vi "ESP301 Home.vi"(5 "Axe Inv":bool, 6 "Input Units":i8(ring) items=["mm", "ps"], 7 "ESP301Ref":T1, 8 "error in":errorcluster, 9 "Axis":i8(ring)=1 items=["Axis 1"=1, "Axis 2"=2, "Axis 3"=3], 11 "VISA Rsrc":refnum<visa-resource-name>="GPIB0::7::INSTR") -> (0 "error out":errorcluster)   [LabVIEW 2019]
uses:
  <userlib>/ESP300/ESP300 GotoState.ctl
  <userlib>/GenProg/WritebyRefNum.vi
panel:
  out "Position":dbl=0.5
  out "Move Done":bool
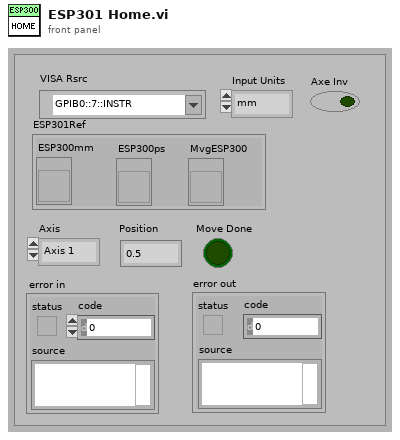
[diagram p1: front panel]
types:
  T1 = cluster{"ESP300mm":refnum<vi>, "ESP300ps":refnum<vi>, "MvgESP300":refnum<vi>}
  T2 = typedef "ESP300 GotoState.ctl" = enum16{"send command", "read position", "check status", "end"}
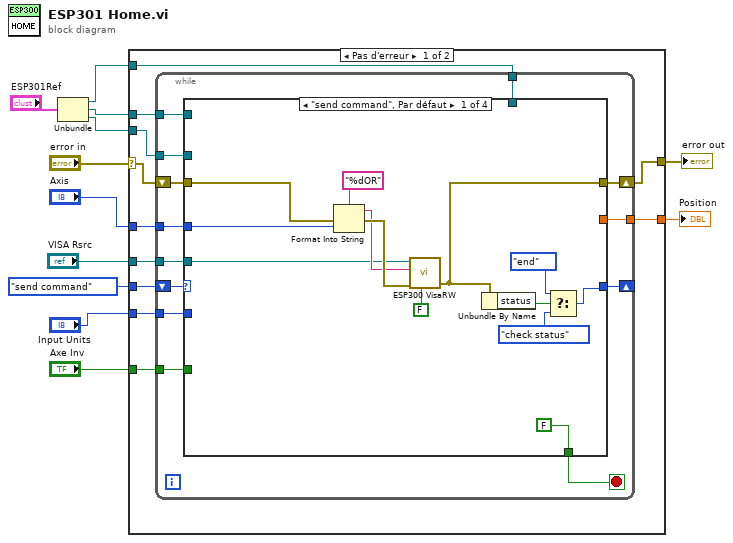
[diagram p0: block diagram]
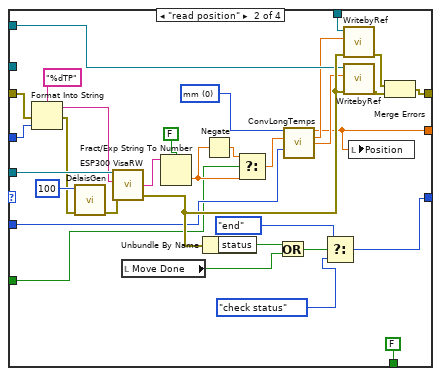
[diagram p2: hidden frame]
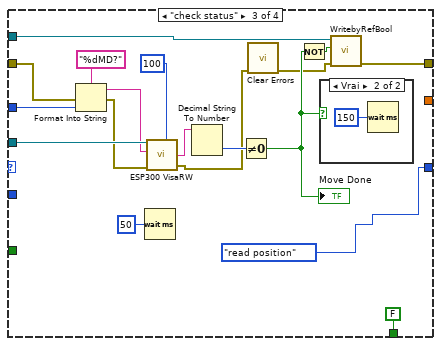
[diagram p3: hidden frame]
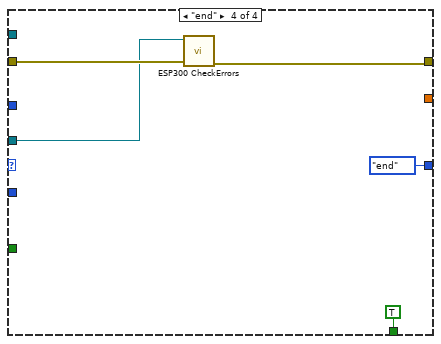
[diagram p5: hidden frame]
diagram:
  n1 = Unbundle("ESP301Ref") -> ("ESP300mm"=w3:refnum<vi>, "ESP300ps"=w5:refnum<vi>, "MvgESP300"=w4:refnum<vi>)
  n2 = case shown="Pas d'erreur" "error in" {
    selector: "error in" -> [w21 w106]
    tunnel: "Axis" -> [w23 _]
    tunnel: [w20 w106] -> w10
    tunnel: ESP300_GotoState."send command" ("Énum") -> [w22 _]
    tunnel: "VISA Rsrc" -> [w19 _]
    tunnel: w4 -> [w18 _]
    tunnel: "Input Units" -> [w17 _]
    tunnel: w3 -> [w16 _]
    tunnel: w5 -> [w15 _]
    tunnel: "Axe Inv" -> [w14 _]
    tunnel: [w13 _] -> w1
    frame No Error {
      n3 = while {
        tunnel: w23 -> [w36]
        shift-right: [w32] -> w20
        shift-left: w21 -> [w34]
        tunnel: w19 -> [w33]
        shift-right: [w30] -> _
        shift-left: w22 -> [w35]
        tunnel: w18 -> [w29]
        tunnel: w17 -> [w28]
        tunnel: w16 -> [w27]
        tunnel: w15 -> [w26]
        tunnel: w14 -> [w25]
        tunnel: [w24] -> w13
        stop <- w31 stop-if-true
        n4 = case shown="\"send command\", Par défaut" w35 {
          tunnel: w36 -> [w48 w79 w97 _]
          tunnel: w34 -> [w47 w78 w96 w103]
          tunnel: w33 -> [w44 w81 w99 w101]
          tunnel: [w41 w62 w87 w102] -> w32
          tunnel: [FALSE FALSE FALSE TRUE] -> w31
          tunnel: [w38 w71 ESP300_GotoState."read position" ("Énum") ESP300_GotoState."end" ("Énum")] -> w30
          tunnel: w29 -> [_ _ w89 _]
          tunnel: w28 -> [_ w55 _ _]
          tunnel: w27 -> [_ w60 _ _]
          tunnel: w26 -> [_ w59 _ _]
          tunnel: w25 -> [_ w51 _ _]
          tunnel: [_ w50 _ _] -> w24
          frame "send command", Default {
            n5 = Format Into String(format string="%dOR", error in=w47, w48) -> (resulting string=w45:string, error out=w46:errorcluster)  [unwired: 1 in]
            n6 = call <userlib>:"ESP300 VisaRW.vi"("Lecture?(T)"=FALSE, "error in (no error)"=w46, "ChaineCom"=w45, "VISA Rsrc"=w44) -> ("error out"=w41:errorcluster)  [unwired: 3 in, 3 out]
            n7 = Unbundle By Name(w41) -> ("status"=w40:bool)
            n8 = Select(t=ESP300_GotoState."end" ("Énum"), s=w40, f=ESP300_GotoState."check status" ("Énum")) -> (s? t:f=w38:T2)
          }
          frame "read position" {
            w58 = i8 0 items=["mm", "ps"] ("Input Units")
            n9 = Format Into String(format string="%dTP", error in=w78, w79) -> (resulting string=w77:string, error out=w66:errorcluster)  [unwired: 1 in]
            n10 = call "DélaisGen.vi"("error in (no error)"=w66, "ms To Wait"=u32 100 ("milliseconds to wait")) -> ("error out"=w67:errorcluster)  [unwired: 9 in]
            n11 = call <userlib>:"ESP300 VisaRW.vi"("error in (no error)"=w67, "ChaineCom"=w77, "VISA Rsrc"=w81) -> ("error out"=w63:errorcluster, "ChaineRep"=w76:string)  [unwired: 4 in, 2 out]
            n12 = local read "Move Done"() -> (w65:bool)
            n13 = Fract/Exp String To Number(use system decimal point (T)=FALSE ("utiliser le séparateur décimal du système (V)"), string=w76) -> (number=w53:dbl)  [unwired: 2 in, 1 out]
            n14 = Unbundle By Name(w63) -> ("status"=w70:bool)
            n15 = Negate(x=w53) -> (-x=w54:dbl)
            n16 = Select(t=w54, s=w51, f=w53) -> (s? t:f=w52:dbl)
            n17 = Or(x=w70, y=w65) -> (x .or. y?=w69:bool)
            n18 = call <userlib>:"ConvLongTemps.vi"("Input Units"=w58, "Units Input"=w52, "Output Units"=w55) -> ("Units Output"=w50:dbl, "Units mm"=w57:dbl, "Units ps"=w56:dbl)  [unwired: 9 in, 1 out]
            n19 = Select(t=ESP300_GotoState."end" ("Énum"), s=w69, f=ESP300_GotoState."check status" ("Énum")) -> (s? t:f=w71:T2)
            n20 = call-poly <userlib>:"WritebyRef.vi"("error in"=w63, "Valeur"=w57, "Control Ref"=w60) -> ("error out"=w61:errorcluster)  [unwired: 8 in]
            n21 = call-poly <userlib>:"WritebyRef.vi"("error in"=w63, "Valeur"=w56, "Control Ref"=w59) -> ("error out"=w64:errorcluster)  [unwired: 8 in]
            n22 = local write "Position"(w50) -> ()
            n23 = Merge Errors(w61, w64) -> (w62:errorcluster)
          }
          frame "check status" {
            n24 = Format Into String(format string="%dMD?", error in=w96, w97) -> (resulting string=w94:string, error out=w95:errorcluster)  [unwired: 1 in]
            n25 = Wait (ms)(milliseconds to wait=u32 50 ("attente (ms)")) -> ()  [unwired: 1 out]
            n26 = call <userlib>:"ESP300 VisaRW.vi"("Délais (0 ms)"=u32 100, "error in (no error)"=w95, "ChaineCom"=w94, "VISA Rsrc"=w99) -> ("error out"=w88:errorcluster, "ChaineRep"=w93:string)  [unwired: 3 in, 2 out]
            n27 = Decimal String To Number(string=w93) -> (number=w91:i32)  [unwired: 2 in, 1 out]
            n28 = Not Equal To 0?(x=w91) -> (x != 0?=w86:bool)
            "Move Done" <- w86
            n29 = call <vilib>:"Clear Errors.vi"("error in (no error)"=w88) -> ("error out"=w83:errorcluster)  [unwired: 5 in, 1 out]
            n30 = Not(x=w86) -> (.not. x?=w85:bool)
            n31 = case shown="Vrai" w86 {
              frame False {
              }
              frame True {
                n32 = Wait (ms)(milliseconds to wait=u32 150) -> ()  [unwired: 1 out]
              }
            }
            n33 = call <userlib>:"WritebyRefBool.vi"("error in"=w83, "Valeur"=w85, "Control Ref"=w89) -> ("error out"=w87:errorcluster)  [unwired: 8 in]
          }
          frame "end" {
            n34 = call <userlib>:"ESP300 CheckErrors.vi"("error in (no error)"=w103, "Ressource VISA In"=w101) -> ("error out"=w102:errorcluster)  [unwired: 4 in, 3 out]
          }
        }
      }
    }
    frame Error {
    }
  }
  "error out" <- w10
  "Position" <- w1
